vi "Run.vi"(7 "Team Index":i32, 8 "Column":i32, 9 "Row":i32, 10 "View":i32[](array[numeric]) caption="View (Team Index, -1: empty)", 11 "Permanent Wall In":refnum<class "Permanent Wall.lvclass">) -> (0 "Replicated":refnum<class "Square.lvclass">, 1 "Direction":T1, 2 "Action":T2, 3 "Square Out":refnum<class "Square.lvclass">)   [LabVIEW 2015, in "Permanent Wall.lvclass"]
uses:
  Permanent Wall.lvclass
  Square/Square.lvclass
  Type Defs/Action Enum.ctl
  Type Defs/Direction Enum.ctl
  Common/Position.ctl
  Permanent Wall.lvclass/Permanent Wall.ctl
  Type Defs/SB Type Defs.lvlib
  Common/Common.lvlib
  Fortress/Fortress.lvclass
panel:
  # "NW\nN\nNE\nE\nSE\nS\nSW\nW"
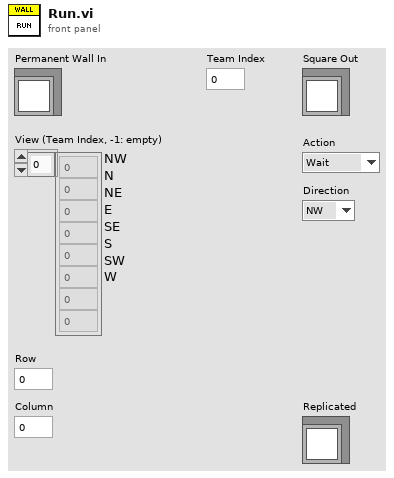
[diagram p1: front panel]
types:
  T1 = typedef "SB Type Defs.lvlib/Direction Enum.ctl" = enum16{"NW", "N", "NE", "E", "SE", "S", "SW", "W"}
  T2 = typedef "SB Type Defs.lvlib/Action Enum.ctl" = enum16{"Wait", "Move", "Attack", "Replicate"}
  T3 = typedef "Common.lvlib/Position.ctl" = cluster{"Column":i32, "Row":i32}
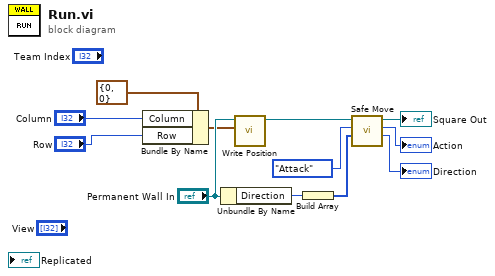
[diagram p0: block diagram]
diagram:
  n1 = Bundle By Name(cluster=T3 {"Column"=0, "Row"=0} ("Position in"), "Column"="Column", "Row"="Row") -> (w1:T3)
  n2 = Unbundle By Name("Permanent Wall In") -> ("Direction"=w3:T1)
  n3 = call-dynamic "Write Position.vi"("Position"=w1, "Fortress in"="Permanent Wall In") -> ("Fortress out"=w8:refnum<class "Permanent Wall.lvclass">)  [unwired: 8 in, 1 out]
  n4 = Build Array(w3) -> (w2:T1[])
  n5 = call "Safe Move.vi"("Directions in"=w2, "Action in"=Action_Enum."Attack" ("Action"), "Fortress In"=w8) -> ("Direction"=→"Direction":T1, "Action out"=→"Action":T2, "Fortress Out"=→"Square Out":refnum<class "Permanent Wall.lvclass">)  [unwired: 5 in, 1 out]
